vi "AssetMgrApplyAssetTemplateResponse_Parse.vi"(8 "error in (no error)":errorcluster, 11 "Message":T17) -> (0 "error out":errorcluster, 1 "Body":T1, 2 "Header":T16, 3 "AssetMgrApplyAssetTemplateResponse":T15)   [LabVIEW 2017]
uses:
  <vilib>/addons/InsightCM/MessageBus/Base/controls/Message.ctl
  <vilib>/addons/InsightCM/MessageBus/Base/controls/MessageHeader.ctl
  <vilib>/addons/InsightCM/MessageBus/Base/controls/KeyValuePair.ctl
  <vilib>/addons/InsightCM/MessageBus/MessageLibrary/AssetManager/controls/AssetMgrApplyAssetTemplateResponse.ctl
  <vilib>/addons/InsightCM/MessageBus/MessageLibrary/AssetManager/controls/AssetMgrApplyAssetTemplateResponseBody.ctl
  <vilib>/addons/InsightCM/MessageBus/Base/controls/AssetNode.ctl
  <vilib>/addons/InsightCM/MessageBus/Base/controls/AssetState.ctl
  <vilib>/addons/InsightCM/MessageBus/Base/controls/AssetNodeSensorGroup.ctl
  <vilib>/addons/InsightCM/MessageBus/Base/controls/WirelessCollectionConfig.ctl
  <vilib>/addons/InsightCM/MessageBus/Base/controls/Condition.ctl
  <vilib>/addons/InsightCM/MessageBus/Base/controls/OperatingState.ctl
  <vilib>/addons/InsightCM/MessageBus/Base/controls/Trigger.ctl
  <vilib>/addons/InsightCM/MessageBus/Base/controls/Metric.ctl
  <vilib>/addons/InsightCM/MessageBus/Base/controls/TrendAlarmRule.ctl
  <vilib>/addons/InsightCM/MessageBus/Base/controls/TrendAlarmLevel.ctl
  <vilib>/addons/InsightCM/MessageBus/Base/controls/AlarmAction.ctl
  <vilib>/addons/InsightCM/MessageBus/Base/controls/AssetNodeReference.ctl
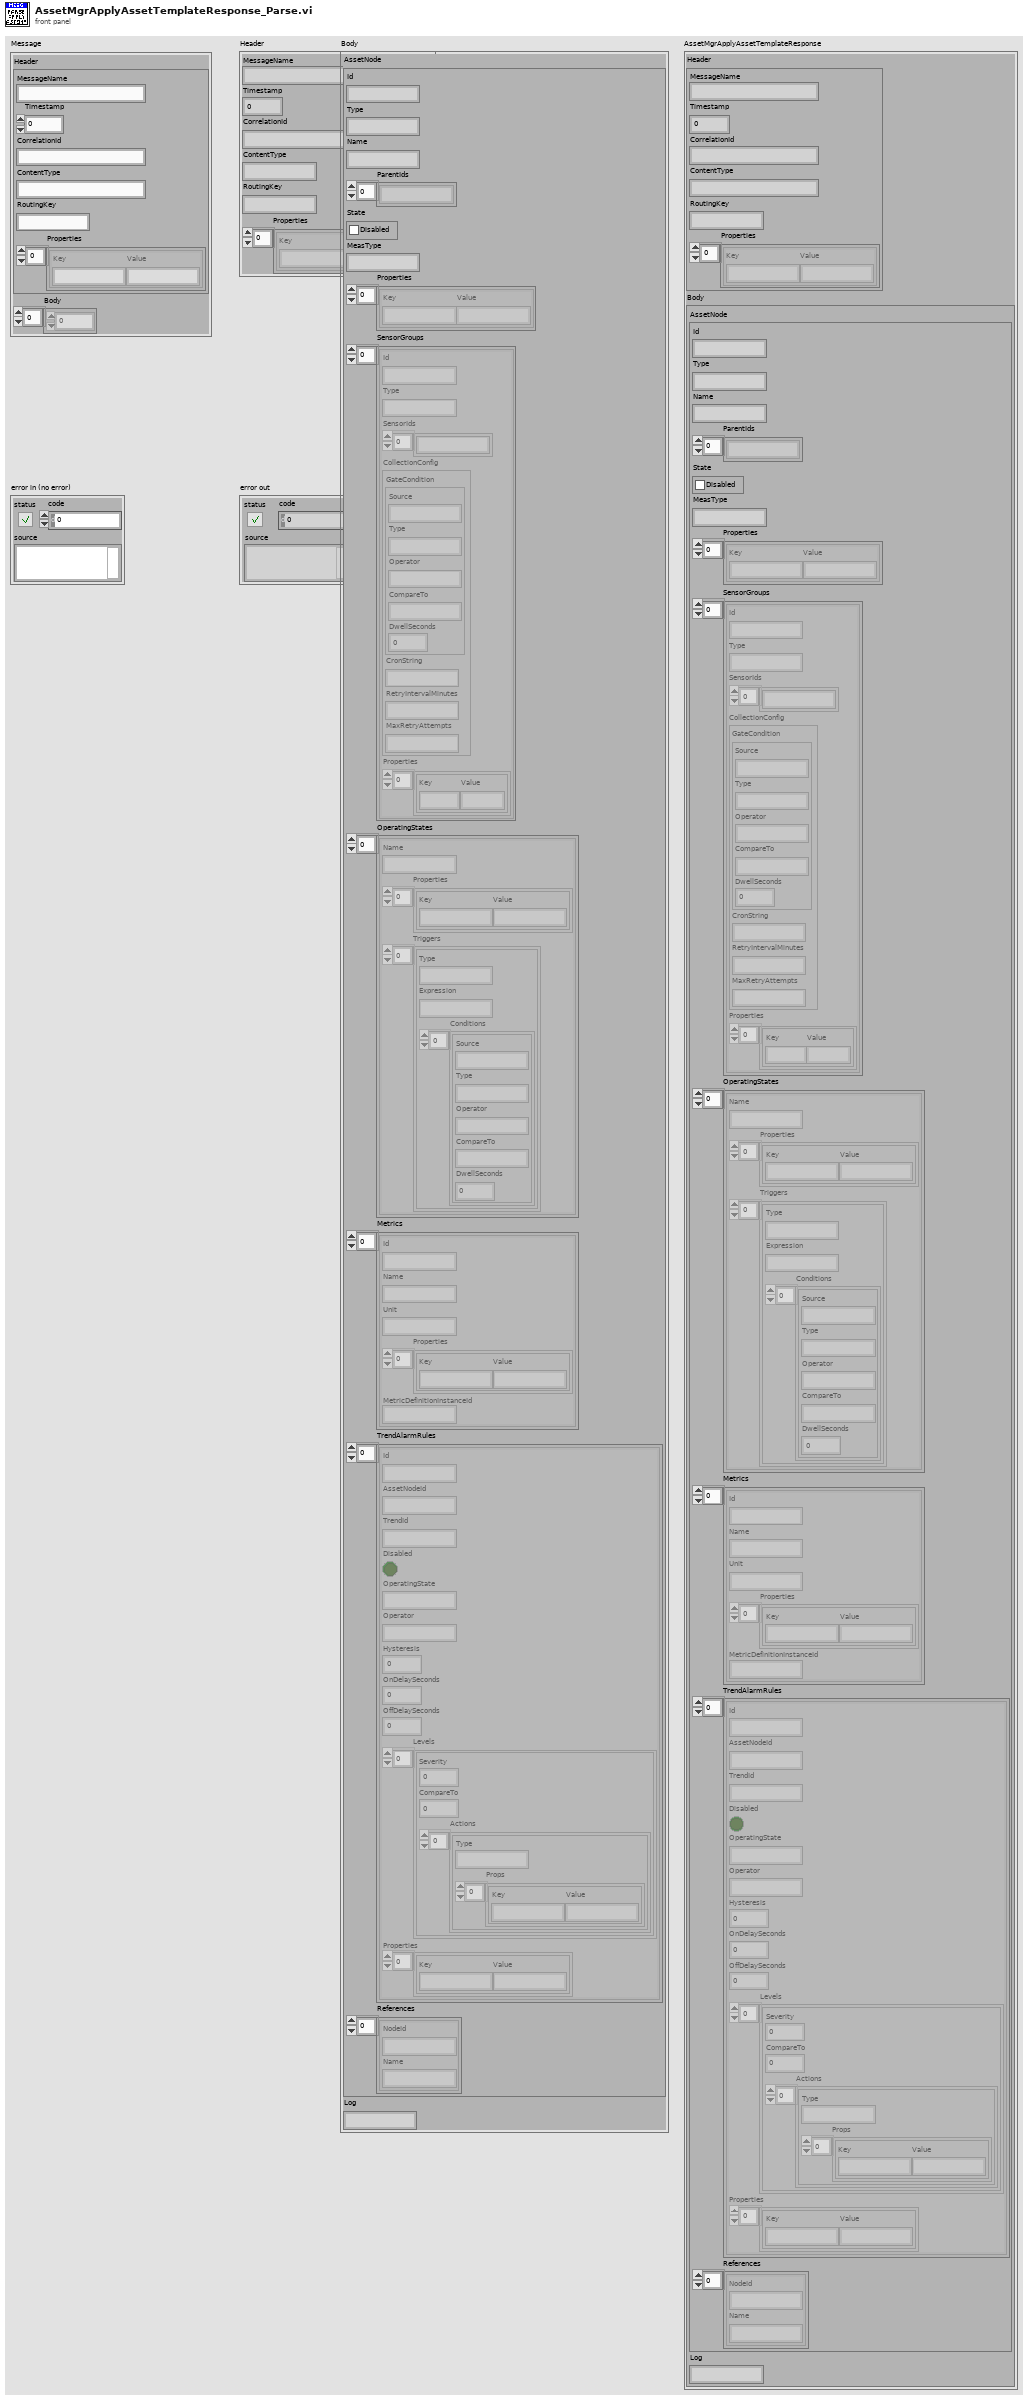
[diagram p1: front panel]
types:
  T1 = typedef "AssetMgrApplyAssetTemplateResponseBody.ctl" = cluster{"AssetNode":T2, "Log":string}
  T2 = typedef "AssetNode.ctl" = cluster{"Id":string, "Type":string, "Name":string, "ParentIds":string[], "State":T3, "MeasType":string, "Properties":T4[], "SensorGroups":T5[], "OperatingStates":T8[], "Metrics":T10[], "TrendAlarmRules":T11[], "References":T14[]}
  T3 = typedef "AssetState.ctl" = cluster{"Disabled":bool}
  T4 = typedef "KeyValuePair.ctl" = cluster{"Key":string, "Value":string}
  T5 = typedef "AssetNodeSensorGroup.ctl" = cluster{"Id":string, "Type":string, "SensorIds":string[], "CollectionConfig":T6, "Properties":T4[]}
  T6 = typedef "WirelessCollectionConfig.ctl" = cluster{"GateCondition":T7, "CronString":string, "RetryIntervalMinutes":string, "MaxRetryAttempts":string}
  T7 = typedef "Condition.ctl" = cluster{"Source":string, "Type":string, "Operator":string, "CompareTo":string, "DwellSeconds":dbl}
  T8 = typedef "OperatingState.ctl" = cluster{"Name":string, "Properties":T4[], "Triggers":T9[]}
  T9 = typedef "Trigger.ctl" = cluster{"Type":string, "Expression":string, "Conditions":T7[]}
  T10 = typedef "Metric.ctl" = cluster{"Id":string, "Name":string, "Unit":string, "Properties":T4[], "MetricDefinitionInstanceId":string}
  T11 = typedef "TrendAlarmRule.ctl" = cluster{"Id":string, "AssetNodeId":string, "TrendId":string, "Disabled":bool, "OperatingState":string, "Operator":string, "Hysteresis":dbl, "OnDelaySeconds":dbl, "OffDelaySeconds":dbl, "Levels":T12[], "Properties":T4[]}
  T12 = typedef "TrendAlarmLevel.ctl" = cluster{"Severity":i32, "CompareTo":dbl, "Actions":T13[]}
  T13 = typedef "AlarmAction.ctl" = cluster{"Type":string, "Props":T4[]}
  T14 = typedef "AssetNodeReference.ctl" = cluster{"NodeId":string, "Name":string}
  T15 = typedef "AssetMgrApplyAssetTemplateResponse.ctl" = cluster{"Header":T16, "Body":T1}
  T16 = typedef "MessageHeader.ctl" = cluster{"MessageName":string, "Timestamp":i64, "CorrelationId":string, "ContentType":string, "RoutingKey":string, "Properties":T4[]}
  T17 = typedef "Message.ctl" = cluster{"Header":T16, "Body":u8[]}
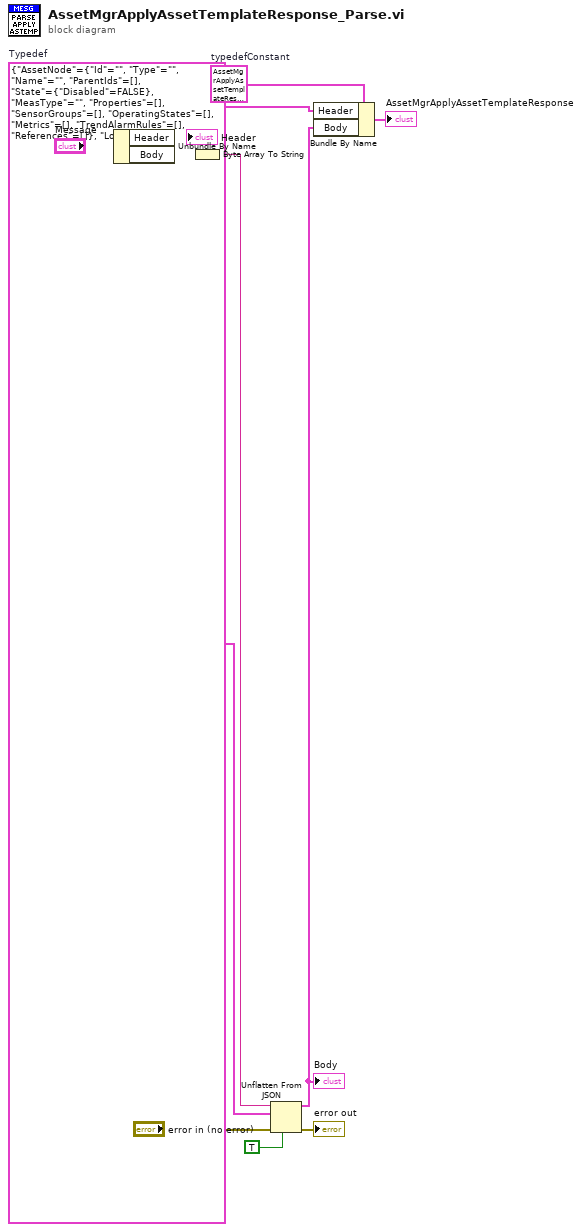
[diagram p0: block diagram]
diagram:
  w3 = T15 {"Header"={"MessageName"="", "Timestamp"=0, "CorrelationId"="", "ContentType"="", "RoutingKey"="", "Properties"=[]}, "Body"={"AssetNode"={"Id"="", "Type"="", "Name"="", "ParentIds"=[], "State"={"Disabled"=FALSE}, "MeasType"="", "Properties"=[], "SensorGroups"=[], "OperatingStates"=[], "Metrics"=[], "TrendAlarmRules"=[], "References"=[]}, "Log"=""}}  # typedefConstant
  w7 = T1 {"AssetNode"={"Id"="", "Type"="", "Name"="", "ParentIds"=[], "State"={"Disabled"=FALSE}, "MeasType"="", "Properties"=[], "SensorGroups"=[], "OperatingStates"=[], "Metrics"=[], "TrendAlarmRules"=[], "References"=[]}, "Log"=""}  # Typedef
  n1 = Unbundle By Name("Message") -> ("Header"=w9:T16, "Body"=w1:u8[])
  "Header" <- w9
  n2 = Byte Array To String(unsigned byte array=w1) -> (string=w6:string)
  n3 = Unflatten From JSON(JSON string=w6, type and defaults=w7, default null elements? (F)=TRUE, error in (no error)="error in (no error)") -> (value=w5:T1, error out=→"error out":errorcluster)  [unwired: 3 in]
  "Body" <- w5
  n4 = Bundle By Name(cluster=w3, "Header"=w9, "Body"=w5) -> (→"AssetMgrApplyAssetTemplateResponse":T15)
